vi "getTravCoordinateSystem.vi"() -> (1 "coordName":string, 2 "Work in Tunnel Coordinates?":T1)   [LabVIEW 2022 SP3]
uses:
  Controls/Tunnel_Coordinates.ctl
  Globals/Meas_global.vi
  Globals/Extra_Commands_Global.vi
  Globals/Trav_pos_global.vi
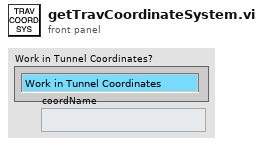
[diagram p1: front panel]
types:
  T1 = typedef "Tunnel_Coordinates.ctl" = enum16{"Work in Tunnel Coordinates", "Work in Model Coordinates"}
  T2 = typedef "Post_Process.ctl" = enum16{"Take New Data", "Post Process Raw Data File"}
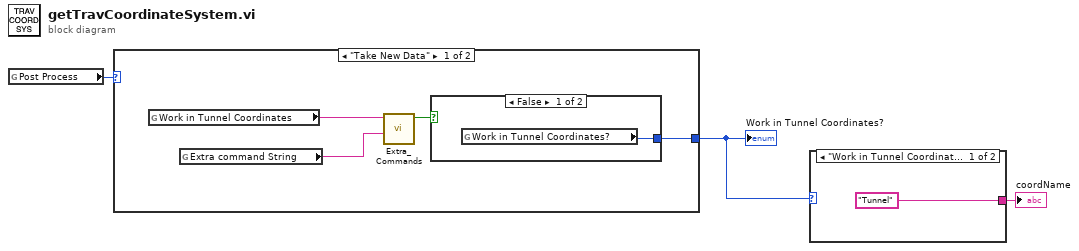
[diagram p0: block diagram]
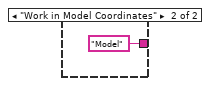
[diagram p2: hidden frame]
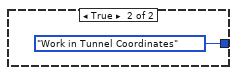
[diagram p3: hidden frame]
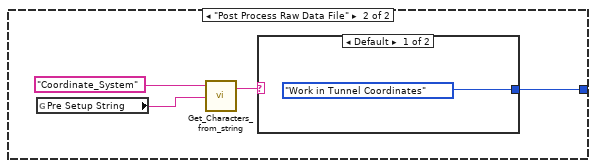
[diagram p4: hidden frame]
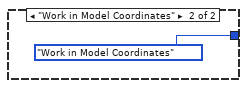
[diagram p5: hidden frame]
diagram:
  n1 = global read "Meas_global.vi" "Post Process"() -> (w3:T2)
  n2 = case shown="\"Take New Data\"" w3 {
    tunnel: [w4 w12] -> w2
    frame "Take New Data" {
      n3 = global read "Extra_Commands_Global.vi" "Work in Tunnel Coordinates"() -> (w7:string)
      n4 = global read "Meas_global.vi" "Extra command String"() -> (w5:string)
      n5 = call "Extra_Commands.vi"("String to Search"=w5, "Command"=w7) -> ("Command Found"=w6:bool)  [unwired: 1 in, 4 out]
      n6 = case shown="False" w6 {
        tunnel: [w8 Tunnel_Coordinates."Work in Tunnel Coordinates" ("Work in Tunnel Coordinates?")] -> w4
        frame False {
          n7 = global read "Trav_pos_global.vi" "Work in Tunnel Coordinates?"() -> (w8:T1)
        }
        frame True {
        }
      }
    }
    frame "Post Process Raw Data File" {
      n8 = global read "Meas_global.vi" "Pre Setup String"() -> (w10:string)
      n9 = call "Get_Characters_from_string.vi"("Input string"=w10, "Variable name"="Coordinate_System" ("Label for characters")) -> ("Value"=w13:string)  [unwired: 1 in, 1 out]
      n10 = case shown="Default" w13 {
        tunnel: [Tunnel_Coordinates."Work in Tunnel Coordinates" ("Work in Tunnel Coordinates?") Tunnel_Coordinates."Work in Model Coordinates" ("Work in Tunnel Coordinates?")] -> w12
        frame Default {
        }
        frame "Work in Model Coordinates" {
        }
      }
    }
  }
  "Work in Tunnel Coordinates?" <- w2
  n11 = case shown="\"Work in Tunnel Coordinates\"" w2 {
    tunnel: ["Tunnel" "Model"] -> w1
    frame "Work in Tunnel Coordinates" {
    }
    frame "Work in Model Coordinates" {
    }
  }
  "coordName" <- w1
